vi "ReaderClose.vi"(8 "NXT":T1={"Hardware"="NXT", "Flattened String"=""}) -> (11 "NXT":T1={"Hardware"="NXT", "Flattened String"=""})   [LabVIEW 2010, in "Packet Recorder.lvlib"]
uses:
  Packet Recorder.lvlib
  <vilib>/NXT/Subs/LVHSConnector.ctl
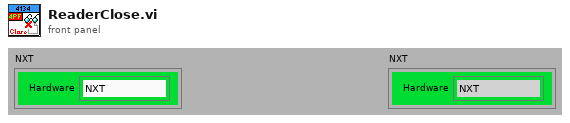
[diagram p1: front panel]
types:
  T1 = typedef "LVHSConnector.ctl" = cluster{"Hardware":string, "Flattened String":string}
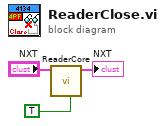
[diagram p0: block diagram]
diagram:
  n1 = call "ReaderCore.vi"("Close"=TRUE, "NXT"="NXT") -> ("NXT"=→"NXT":T1)  [unwired: 9 in]
